vi "Write Size.vi"(8 "error in (no error)":errorcluster, 10 "Size":cluster{"Width":u16, "Height":u16}, 11 "Bitmap Canvas in":refnum<class "Bitmap Canvas.lvclass">) -> (0 "error out":errorcluster, 3 "Bitmap Canvas out":refnum<class "Bitmap Canvas.lvclass">)   [LabVIEW 2023, in "Font Glyph Drawer Interface.lvlib" / "Bitmap Canvas.lvclass"]
uses:
  Bitmap Canvas.lvclass
  Bitmap Canvas.lvclass/Bitmap Canvas.ctl
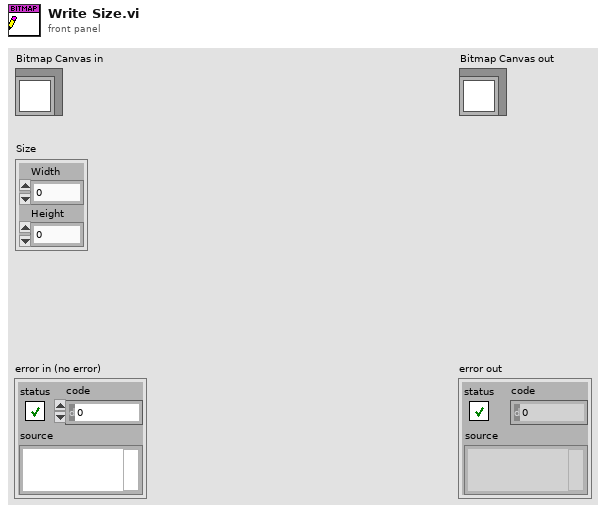
[diagram p1: front panel]
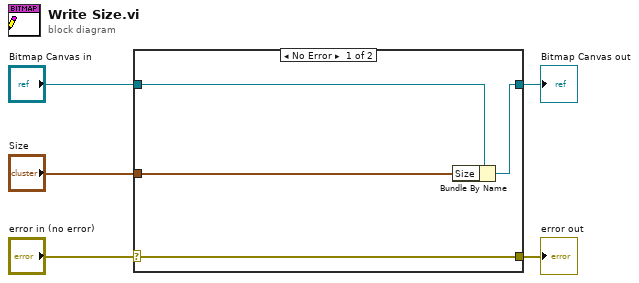
[diagram p0: block diagram]
diagram:
  n1 = case shown="No Error" "error in (no error)" {
    selector: "error in (no error)" -> [w9 w10]
    tunnel: [w9 w10] -> w4
    tunnel: [w7 w11] -> w2
    tunnel: "Bitmap Canvas in" -> [w8 w11]
    tunnel: "Size" -> [w6 _]
    frame No Error {
      n2 = Bundle By Name(cluster=w8, "Size"=w6) -> (w7:refnum<class "Bitmap Canvas.lvclass">)
    }
    frame Error {
    }
  }
  "error out" <- w4
  "Bitmap Canvas out" <- w2
